vi "Record_Initialization_1D.vi"(0 "Indexed Names":string[](array[string]), 1 "Refnum in":refnum<k34>, 2 "Period":i64, 3 "Buffer size":i64, 5 "Indexed SV Refnums":refnum<k21>[](array[refnum]), 7 "Indexed Type Code":i32[](array[numeric]), 11 "error in (no error)":errorcluster) -> (4 "Array of sizes":i32[](array[numeric]), 6 "Array of channel names":string[][](array[string]), 8 "Array of 1D waveforms":waveform(dbl)[][](array[waveform]), 15 "error out":errorcluster)   [LabVIEW 2014]
doc: "<B>Copyright</B>: (c) MHWirth 2015. All rights are reserved.\n\nThis subVI sets the properties of the TDMS file for recording <B>1D arrays</B>, and prepares the name of channels for each group.\n\nEvery 1D array is saved in one group (sheet), and each element is saved in one channel (column)."
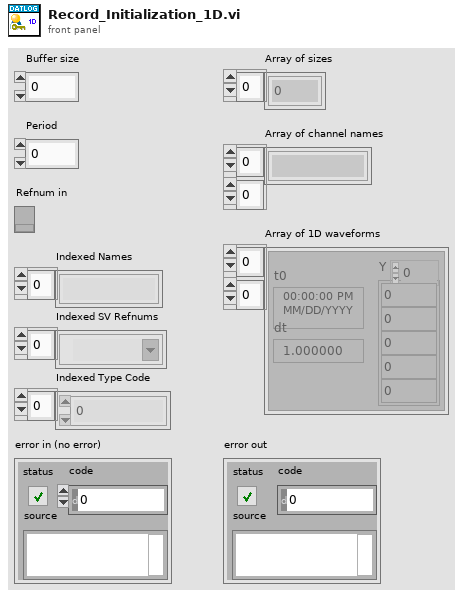
[diagram p1: front panel]
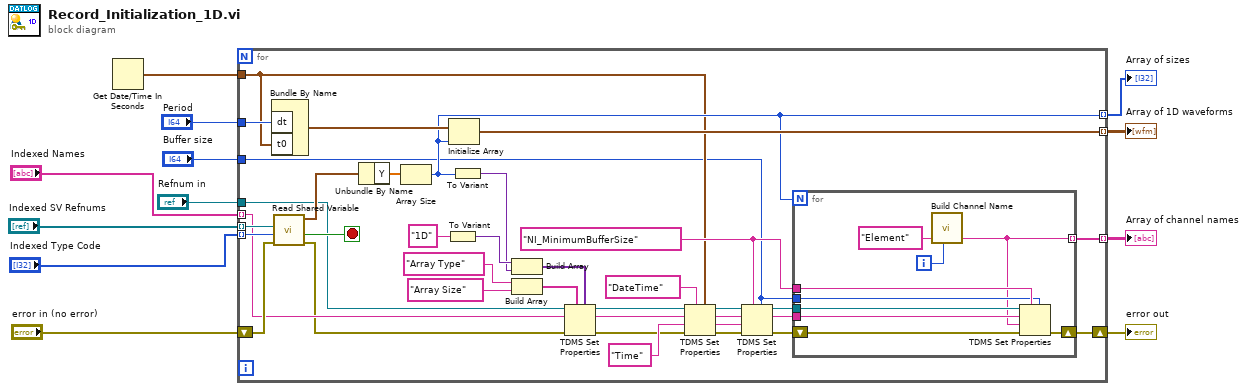
[diagram p0: block diagram]
diagram:
  n1 = Get Date/Time In Seconds() -> (seconds since 1Jan1904=w1:timestamp)
  n2 = for {
    tunnel: "Indexed Names" -> [w33] mode=indexing
    tunnel: "Indexed Type Code" -> [w47] mode=indexing
    tunnel: "Indexed SV Refnums" -> [w48] mode=indexing
    tunnel: "Refnum in" -> [w34]
    shift-right: [w20] -> w8
    shift-left: "error in (no error)" -> [w49]
    tunnel: "Buffer size" -> [w13]
    tunnel: [w15] -> w12 mode=indexing
    tunnel: w1 -> [w14]
    tunnel: "Period" -> [w27]
    tunnel: [w25] -> w11 mode=indexing
    tunnel: [w17] -> w10 mode=indexing
    stop <- w46 stop-if-true
    w16 = "NI_MinimumBufferSize"
    n3 = Bundle By Name("dt"=w27, "t0"=w14) -> (w26:waveform(dbl))  [unwired: 1 in]
    n4 = call "Read Shared Variable.vi"("Error In"=w49, "Type code"=w47, "Refnum"=w48) -> ("Error Out"=w32:errorcluster, "status"=w46:bool, "Waveform out"=w45:waveform(dbl))  [unwired: 5 in, 1 out]
    n5 = Unbundle By Name(w45) -> ("Y"=w44:dbl[])
    n6 = Array Size(array=w44) -> (size(s)=w15:i32)
    n7 = To Variant(anything="1D") -> (Variant=w30:variant)
    n8 = Initialize Array(w26, w15) -> (w25:waveform(dbl)[])
    n9 = To Variant(anything=w15) -> (Variant=w29:variant)
    n10 = Build Array(w30, w29) -> (w28:variant[])
    n11 = Build Array("Array Type", "Array Size") -> (w35:string[])
    n12 = TDMS Set Properties(5:w28, 7:w35, 8:w32, 10:w33, 11:w34) -> (0:w22:errorcluster, 2:w23:string, 3:w24:refnum<k34>)  [unwired: 1 in, 1 out]
    n13 = TDMS Set Properties(5:w14, 7:"DateTime" ("property names"), 8:w22, 9:"Time", 10:w23, 11:w24) -> (0:w43:errorcluster, 1:w42:string, 2:w41:string, 3:w40:refnum<k34>)
    n14 = TDMS Set Properties(5:w13, 7:w16, 8:w43, 9:w42, 10:w41, 11:w40) -> (0:w21:errorcluster, 2:w18:string, 3:w19:refnum<k34>)  [unwired: 1 out]
    n15 = for {
      N: w15 -> [_]
      tunnel: [w50] -> w17 mode=indexing
      shift-right: [w57] -> w20
      shift-left: w21 -> [w58]
      tunnel: w19 -> [w56]
      tunnel: w18 -> [w55]
      tunnel: w16 -> [w54]
      tunnel: w13 -> [w53]
      i -> [w52]
      n16 = call "Build Channel Name.vi"("String in"="Element", "Numeric"=w52) -> ("String out"=w50:string)  [unwired: 7 in]
      n17 = TDMS Set Properties(5:w53, 7:w54, 8:w58, 9:w50, 10:w55, 11:w56) -> (0:w57:errorcluster)  [unwired: 3 out]
    }
  }
  "Array of sizes" <- w12
  "Array of 1D waveforms" <- w11
  "Array of channel names" <- w10
  "error out" <- w8
